vi "Change Currency.vi"(11 "Coin":cluster{"Denomination":string, "Value":dbl}[](array[cluster])) -> (0 "error out":errorcluster)   [LabVIEW 2020, in "Config File Management.lvlib"]
doc: "Writes the New Currency Configuration into the Config File."
uses:
  Config File Management.lvlib
  <vilib>/Utility/config.llb/Write Key (String).vi
  <vilib>/Utility/config.llb/Write Key (Double).vi
  <vilib>/Utility/config.llb/NI_LVConfig.lvlib
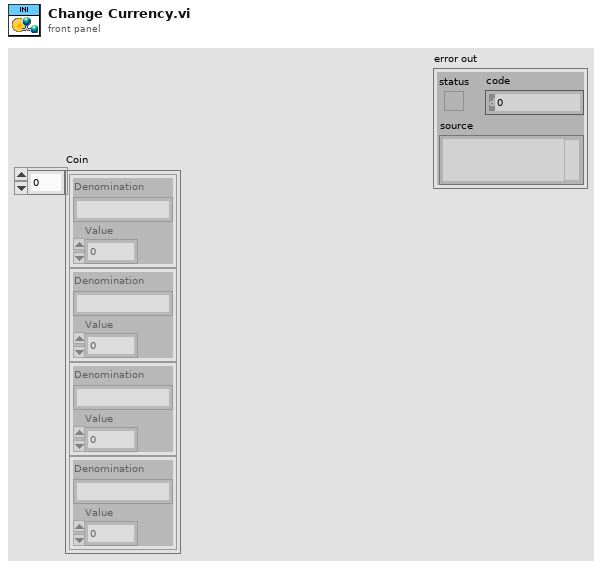
[diagram p1: front panel]
types:
  T1 = typedef "NI_LVConfig.lvlib/Config Data RefNum.ctl" = refnum<k1>
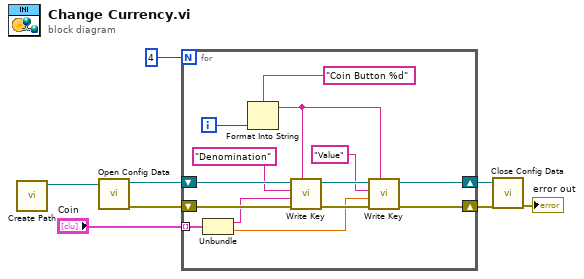
[diagram p0: block diagram]
diagram:
  n1 = call "Create Path.vi"() -> ("Config File path"=w4:path)  [unwired: 11 in]
  n2 = call <vilib>:"Open Config Data.vi"("configuration file path"=w4) -> ("error out"=w8:errorcluster, "refnum"=w7:T1)  [unwired: 8 in, 1 out]
  n3 = for {
    N: 4 -> [_]
    shift-right: [w19] -> w5
    shift-left: w8 -> [w22]
    shift-right: [w16] -> w6
    shift-left: w7 -> [w21]
    tunnel: "Coin" -> [w12] mode=indexing
    i -> [w9]
    n4 = Unbundle(w12) -> ("Denomination"=w11:string, "Value"=w10:dbl)
    n5 = Format Into String(format string="Coin Button %d", w9) -> (resulting string=w15:string)  [unwired: 2 in, 1 out]
    n6 = call-poly <vilib>:"Write Key.vi"("section"=w15, "error in (no error)"=w22, "value"=w11, "key"="Denomination", "refnum"=w21) -> ("error out"=w18:errorcluster, "refnum out"=w17:T1)  [unwired: 4 in, 1 out]
    n7 = call-poly <vilib>:"Write Key.vi"("section"=w15, "error in (no error)"=w18, "value"=w10, "key"="Value", "refnum"=w17) -> ("error out"=w19:errorcluster, "refnum out"=w16:T1)  [unwired: 4 in, 1 out]
  }
  n8 = call <vilib>:"Close Config Data.vi"("error in (no error)"=w5, "refnum"=w6) -> ("error out"=→"error out":errorcluster)  [unwired: 8 in, 1 out]
